vi "UpdateOnExitOpState.vi"(8 "error in (no error)":errorcluster, 9 "operating state":string, 10 "data group":string, 11 "open data event configs in":variant) -> (0 "error out":errorcluster, 3 "open data event configs out":variant)   [LabVIEW 2017, in "DataEventCreator.lvlib"]
uses:
  <vilib>/addons/InsightCM/Devices/Shared/Common/DataEventCreator/DataEventCreator.lvlib
  <vilib>/addons/InsightCM/Devices/Shared/Cms/CmsDataEventCreator/controls/DataEventConfig.ctl
  <vilib>/addons/InsightCM/Devices/Shared/Cms/CmsDataEventCreator/controls/AcqParams.ctl
  <vilib>/addons/InsightCM/Devices/Shared/Common/DataAccumulator/controls/AccumulationSettings.ctl
  <vilib>/addons/InsightCM/Devices/Shared/Common/DataAccumulator/controls/accumulationType.ctl
  <vilib>/addons/InsightCM/Devices/Shared/Common/DVRBuffer/controls/BufferLocation.ctl
  <vilib>/addons/PointValueMap/controls/PointMap.ctl
  <vilib>/addons/InsightCM/Devices/Shared/Cms/CmsDataEventCreator/CmsDataEventCreator.lvlib
  <vilib>/addons/PointValueMap/PointValueMap.lvlib
  <vilib>/addons/InsightCM/Devices/Shared/Common/DVRBuffer/DVRBuffer.lvlib
  <vilib>/addons/InsightCM/Devices/Shared/Common/DataAccumulator/DataAccumulator.lvlib
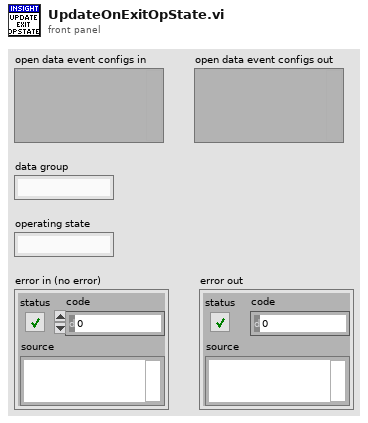
[diagram p1: front panel]
types:
  T1 = typedef "CmsDataEventCreator.lvlib/DataEventConfig.ctl" = cluster{"AcqParams":T2, "OpState":string, "ExitOpState":bool, "Reason":string, "StreamId":string, "Map":T6, "DataSetIds":variant, "IncludeWaveforms":bool, "TrendPointsOnly":bool}
  T2 = typedef "CmsDataEventCreator.lvlib/AcqParams.ctl" = cluster{"Stream":bool, "PreTrigger":i32, "CollectOnEnter":bool, "Enter PreTrigger":i32, "Enter Length":dbl, "CollectOnExit":bool, "ContinuousData":bool, "Accumulation Settings":T3}
  T3 = typedef "DataAccumulator.lvlib/AccumulationSettings.ctl" = cluster{"Type":T4, "Length":dbl, "Max Time (sec)":dbl, "Start Block":T5, "Acquired (sec)":dbl, "Acquired (pulses)":i32, "Initial Pulse Offset":dbl, "Stop Block":T5, "LastBlockAdded":u32}
  T4 = typedef "DataAccumulator.lvlib/accumulationType.ctl" = enum16{"none", "seconds", "revolutions"}
  T5 = typedef "DVRBuffer.lvlib/BufferLocation.ctl" = cluster{"Block":u32, "Index":i32}
  T6 = typedef "PointValueMap.lvlib/PointMap.ctl" = refnum<data-value>
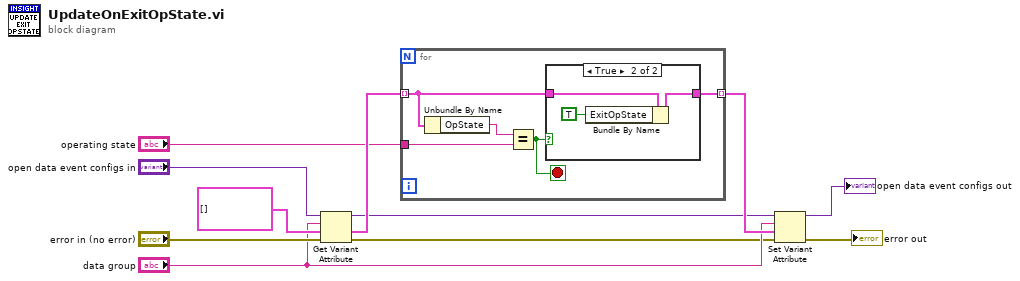
[diagram p0: block diagram]
diagram:
  n1 = Get Variant Attribute(Variant="open data event configs in", name="data group", default value (empty Variant)=T1[] [], error in="error in (no error)") -> (duplicate Variant=w1:variant, value=w11:T1[], error out=w2:errorcluster)  [unwired: 1 out]
  n2 = for {
    tunnel: w11 -> [w14] mode=indexing
    tunnel: "operating state" -> [w15]
    tunnel: [w13] -> w9 mode=indexing
    stop <- w12 stop-if-true
    n3 = Unbundle By Name(w14) -> ("OpState"=w16:string)
    n4 = Equal?(x=w16, y=w15) -> (x = y?=w12:bool)
    n5 = case shown="True" w12 {
      tunnel: w14 -> [w17 w20]
      tunnel: [w17 w18] -> w13
      frame False {
      }
      frame True {
        n6 = Bundle By Name(cluster=w20, "ExitOpState"=TRUE) -> (w18:T1)
      }
    }
  }
  n7 = Set Variant Attribute(Variant=w1, name="data group", value=w9, error in=w2) -> (Variant out=→"open data event configs out":variant, error out=→"error out":errorcluster)  [unwired: 1 out]
